vi "DotNETCam_ClassCast.vi"(11 "DotNETCamIn":refnum<class>) -> (3 "DotNETCamOut":refnum<class "DotNETCam.lvclass">)   [LabVIEW 2021, in "DotNETCam.lvclass"]
uses:
  DotNETCam.lvclass
  DotNETCam.lvclass/DotNETCam.ctl
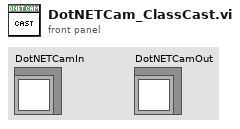
[diagram p1: front panel]
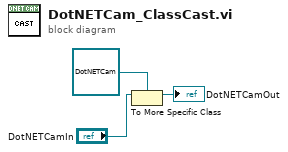
[diagram p0: block diagram]
diagram:
  n1 = To More Specific Class(target class=refnum<class "DotNETCam.lvclass"> refnum ("reference in"), reference="DotNETCamIn") -> (specific class reference=→"DotNETCamOut":refnum<class "DotNETCam.lvclass">)  [unwired: 1 in, 1 out]
